vi "xyz-ast_express.vi"(0 "Image":dbl[][](array[numeric]), 1 "FFT":T2, 2 "Sizes":T1, 5 "R":dbl, 9 "Threshold type":u16(ring) items=["Top fraction", "Top value"], 11 "Threshold":dbl=2.0, 12 "FFT allocated?":bool=TRUE, 13 "Positive angle":dbl) -> (4 "XYZ":dbl[](array[numeric]), 6 "G":dbl[][](graph), 8 "Gx":dbl[][](graph), 10 "Gy":dbl[][](graph), 14 "dR":dbl[](array[numeric]), 15 "Filtered G":dbl[][](graph))   [LabVIEW 2015]
doc: "Single vi for calculating XYZ position of the particle.\n\nINPUT\nImage - input image\nR - radius of the window (should be >0.5)\nThreshold type, - type of threshold to apply:\n \"Top fraction\" - sets threshold as max_intensity/Threshold, e.g., for a Threshold=2 the threshold will be set to half the maximum pixel value \n \"Top value\" - sets the threshold to Threshold\nThreshold - threshold value\nFFT allocated? - must be set to true (default) if FFT and Sizes are connected. If set to False, FFT and Sizes inputs are ignored\nFFT, Sizes - Fourier transforms and sizes obtained from Local gradient preallocation\nPositive angle - angle in degrees that defines orientation of the image of the particle which corresponds to positive z-value\n\nOUTPUT\nXYZ - x,y position of the particle in pixels (for original image), z-value\nFiltered G - filtered local gradient magnitude image\nG,Gx,Gy - magnitude, horizontal and vertical local gradients correspondingly.\ndR - distance from the center to each line (1D vector)\n\nAuthor: Anatolii Kashchuk"
panel:
  in  "Weights type":u16(ring)=1 items=["None", "G", "G^2"]
  # "Author: Anatolii Kashchuk"
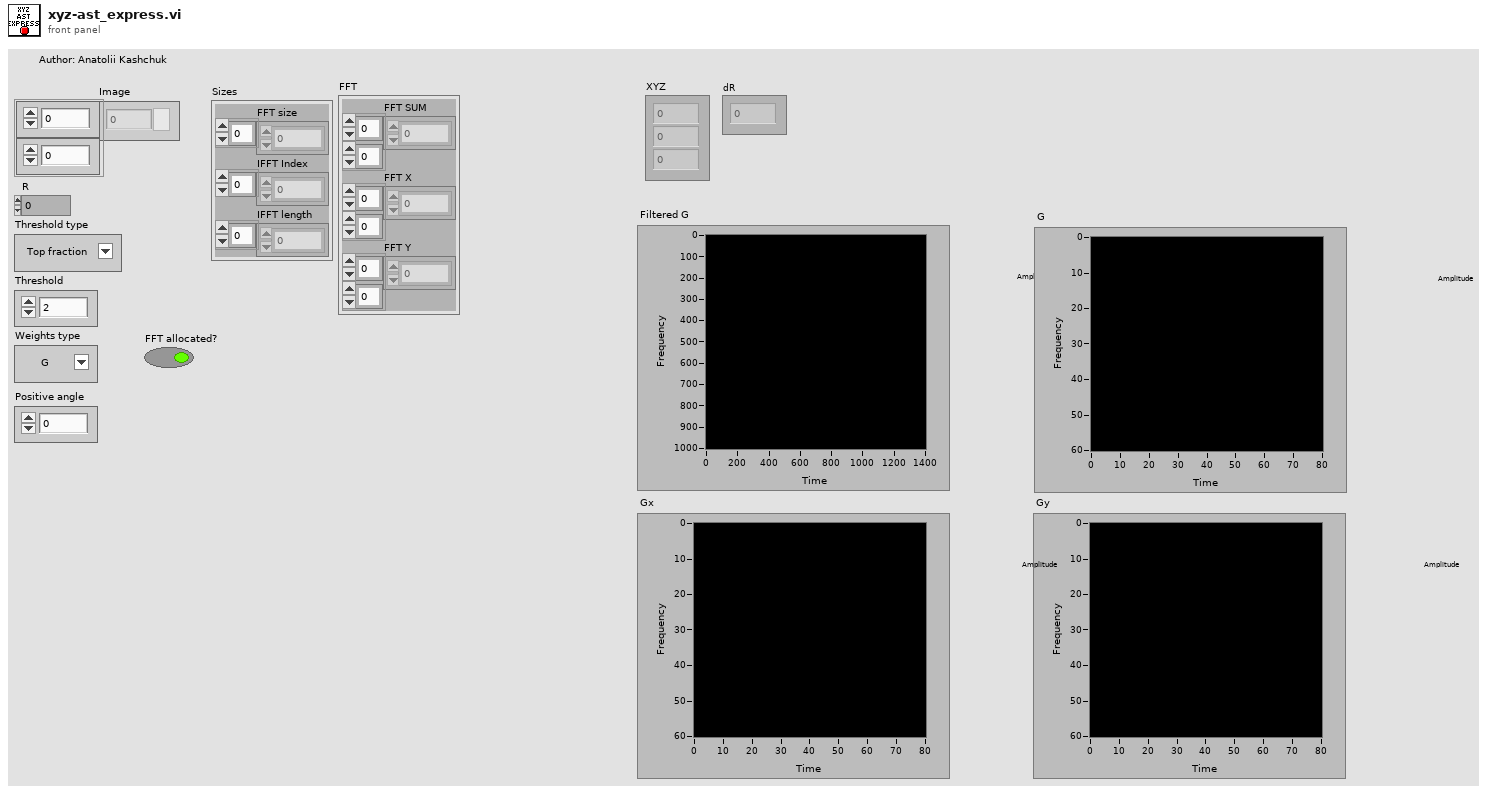
[diagram p1: front panel]
types:
  T1 = cluster{"FFT size":u32[], "IFFT Index":i32[], "IFFT length":u32[]}
  T2 = cluster{"FFT SUM":cdb[][], "FFT X":cdb[][], "FFT Y":cdb[][]}
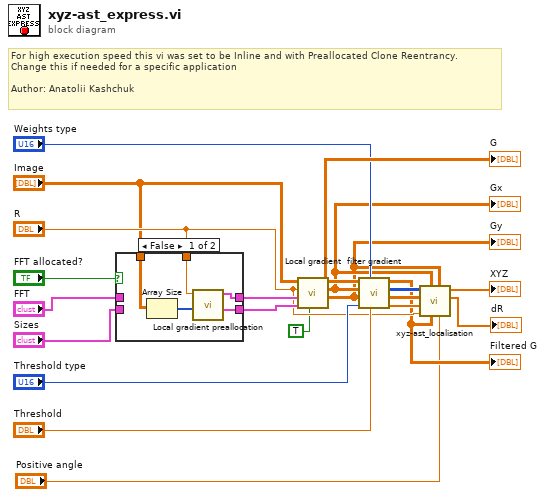
[diagram p0: block diagram]
diagram:
  # "For high execution speed this vi was set to be Inline and with Preallocated Clone Reentrancy. \nChange this if needed for a specific application\n\nAuthor: Anatolii Kashchuk"
  n1 = case shown="False" "FFT allocated?" {
    tunnel: [w26 w28] -> w18
    tunnel: [w25 w27] -> w17
    tunnel: "FFT" -> [_ w28]
    tunnel: "Sizes" -> [_ w27]
    tunnel: "R" -> [w24 _]
    tunnel: "Image" -> [w22 _]
    frame False {
      n2 = Array Size(array=w22) -> (size(s)=w23:i32[])
      n3 = call "Local gradient preallocation.vi"("Image size"=w23, "R"=w24) -> ("Sizes"=w25:T1, "FFT"=w26:T2)  [unwired: 8 in]
    }
    frame True {
    }
  }
  n4 = call "Local gradient.vi"("FFT allocated?"=TRUE, "Sizes"=w17, "FFT"=w18, "R"="R", "Image"="Image") -> ("Gy"=w9:dbl[][], "Gx"=w10:dbl[][], "G"=w21:dbl[][])  [unwired: 4 in]
  "Gy" <- w9
  "Gx" <- w10
  "G" <- w21
  n5 = call "filter gradient.vi"("Threshold"="Threshold", "Weights type"="Weights type", "Threshold type"="Threshold type", "Gy"=w9, "Gx"=w10, "G"=w21) -> ("Weights"=w11:dbl[], "gradients"=w12:dbl[][], "centers"=w13:i32[][], "Filtered G"=w3:dbl[][])  [unwired: 2 out]
  "Filtered G" <- w3
  n6 = call "xyz-ast_localisation.vi"("Positive angle"="Positive angle", "Gy"=w9, "Gthr"=w3, "Gx"=w10, "R"="R", "weights"=w11, "B points"=w12, "A points"=w13) -> ("dR"=→"dR":dbl[], "XYZ"=→"XYZ":dbl[])  [unwired: 2 in]
